vi "complex_to_string.vi"(11 "Numeric":cdb format="%#_13g") -> (3 "output string":string)   [LabVIEW 2014]
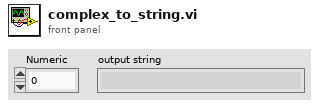
[diagram p1: front panel]
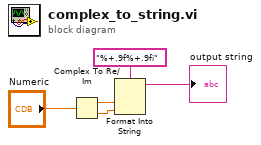
[diagram p0: block diagram]
diagram:
  n1 = Complex To Re/Im(x + iy="Numeric") -> (x=w2:dbl, y=w1:dbl)
  n2 = Format Into String(format string="%+.9f%+.9fi", w2, w1) -> (resulting string=→"output string":string)  [unwired: 2 in, 1 out]
